vi "CK_CameraParse URL.vi"(10 "Full":bool, 11 "CameraIP":string) -> (0 "cgi string":string, 1 "parameters":T1(array[cluster]), 2 "port":i32, 3 "address":string)   [LabVIEW 2017]
panel:
  # "http://roboRIO-419-FRC.local:5800/?action=stream"
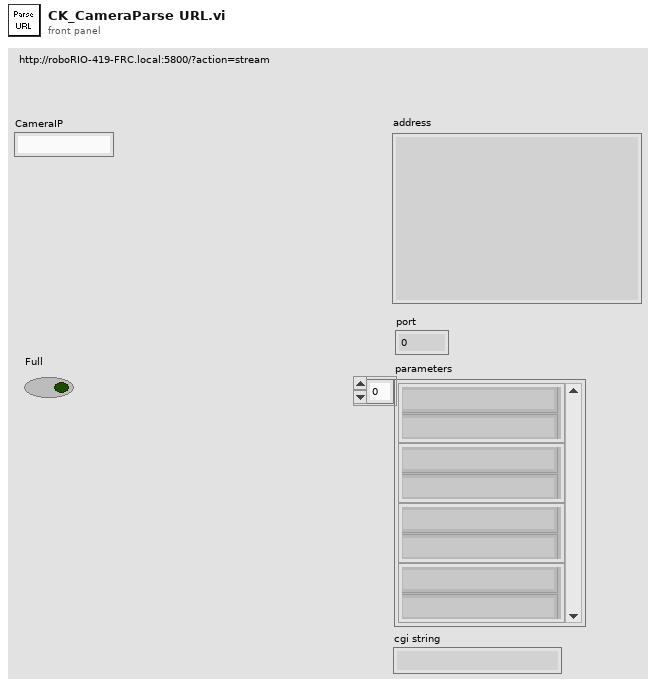
[diagram p1: front panel]
types:
  T1 = cluster{"token string":string, "token string 2":string}[]
  T2 = cluster{"token string":string, "offset past token":i32}
  T3 = cluster{"token string":string, "offset past token":i32}[]
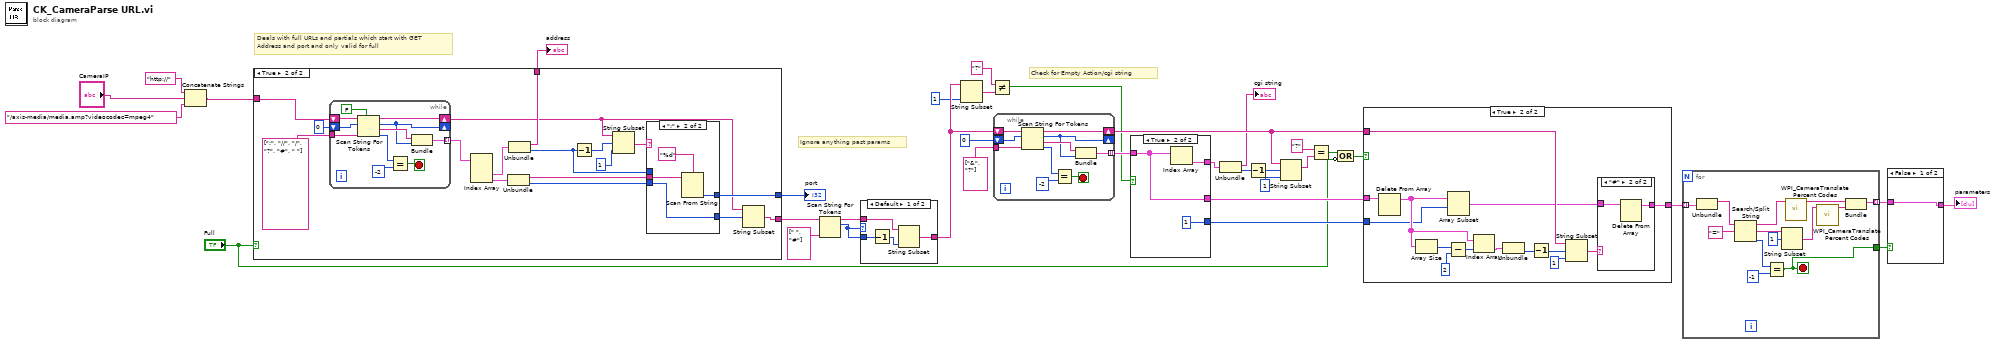
[diagram p0: block diagram]
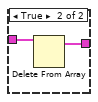
[diagram p4: hidden frame]
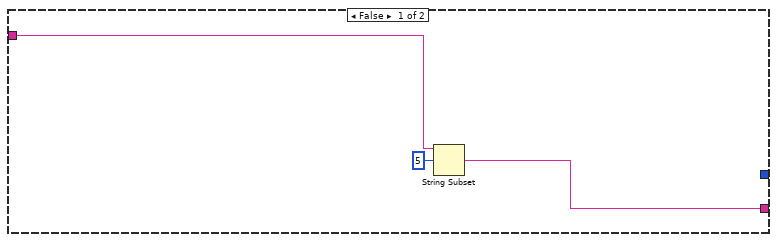
[diagram p5: hidden frame]
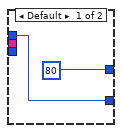
[diagram p6: hidden frame]
diagram:
  # "Check for Empty Action/cgi string"
  # "Ignore anything past params"
  # "Deals with full URLs and partials which start with GET \nAddress and port and only valid for full"
  n1 = Concatenate Strings("http://" ("string"), "CameraIP", "/axis-media/media.amp?videocodec=mpeg4" ("string")) -> (w2:string)
  n2 = case shown="True" "Full" {
    tunnel: [_ w50] -> w35
    tunnel: [_ w49] -> w34
    tunnel: w2 -> [w38 w45]
    tunnel: [w37 w44] -> w16
    frame False {
      n3 = String Subset(string=w38, offset (0)=5) -> (substring=w37:string)  [unwired: 1 in]
    }
    frame True {
      n4 = while {
        tunnel: string[] [":", "//", "/", "?", "#", " "] -> [w72]
        shift-right: [w70] -> w46
        shift-left: w45 -> [w71]
        shift-right: [w63] -> _
        shift-left: 0 ("offset past token") -> [w69]
        tunnel: [w64] -> w53 mode=indexing
        stop <- w67 stop-if-true
        n5 = Scan String For Tokens(5:FALSE ("allow empty tokens? (F)"), 6:w72, 8:w69, 9:w71) -> (0:w65:i32, 1:w66:string, 2:w63:i32, 3:w70:string)  [unwired: 2 in]
        n6 = Equal?(x=w65, y=-2) -> (x = y?=w67:bool)
        n7 = Bundle("token string"=w66, "offset past token"=w63) -> (w64:T2)  [unwired: 1 in]
      }
      n8 = Index Array(array=w53) -> (element #2=w52:T2, element #3=w51:T2)  [unwired: 3 in, 1 out]
      n9 = Unbundle(w51) -> ("token string"=w43:string, "offset past token"=w48:i32)
      n10 = Unbundle(w52) -> ("token string"=w49:string, "offset past token"=w47:i32)
      n11 = Decrement(x=w47) -> (x-1=w41:i32)
      n12 = String Subset(string=w46, offset (0)=w41, length (rest)=1) -> (substring=w40:string)
      n13 = case shown="\":\"" w40 {
        tunnel: w43 -> [_ w61]
        tunnel: [80 w59] -> w50
        tunnel: w48 -> [_ w58]
        tunnel: [w56 w58] -> w39
        tunnel: w47 -> [w56 _]
        frame Default {
        }
        frame ":" {
          n14 = Scan From String(format string="%d", input string=w61) -> (output 1=w59:i32)  [unwired: 3 in, 3 out]
        }
      }
      n15 = String Subset(string=w46, offset (0)=w39) -> (substring=w44:string)  [unwired: 1 in]
    }
  }
  "address" <- w34
  "port" <- w35
  n16 = Scan String For Tokens(6:string[] [" ", "#"], 9:w16) -> (2:w13:i32, 3:w14:string)  [unwired: 4 in, 2 out]
  n17 = case shown="Default" w13 {
    tunnel: w13 -> [w74 _]
    tunnel: [w75 w77] -> w12
    tunnel: w14 -> [w76 w77]
    frame Default {
      n18 = Decrement(x=w74) -> (x-1=w73:i32)
      n19 = String Subset(string=w76, length (rest)=w73) -> (substring=w75:string)  [unwired: 1 in]
    }
    frame -2, -1 {
    }
  }
  n20 = String Subset(string=w12, length (rest)=1 ("length (rest)")) -> (substring=w10:string)  [unwired: 1 in]
  n21 = Not Equal?(x="?" ("format string"), y=w10) -> (x != y?=w7:bool)
  n22 = while {
    tunnel: string[] ["&", "?"] -> [w87]
    shift-right: [w85] -> w27
    shift-left: w12 -> [w86]
    shift-right: [w78] -> _
    shift-left: 0 ("offset past token") -> [w84]
    tunnel: [w79] -> w28 mode=indexing
    stop <- w82 stop-if-true
    n23 = Scan String For Tokens(6:w87, 8:w84, 9:w86) -> (0:w80:i32, 1:w81:string, 2:w78:i32, 3:w85:string)  [unwired: 3 in]
    n24 = Equal?(x=w80, y=-2) -> (x = y?=w82:bool)
    n25 = Bundle("token string"=w81, "offset past token"=w78) -> (w79:T2)  [unwired: 1 in]
  }
  n26 = case shown="True" w7 {
    tunnel: w28 -> [w88 w90]
    tunnel: [_ w91] -> w25
    tunnel: [w88 w90] -> w8
    tunnel: [_ 1] -> w6
    frame False {
    }
    frame True {
      n27 = Index Array(array=w90) -> (element=w91:T2)  [unwired: 1 in]
    }
  }
  n28 = Unbundle(w25) -> ("token string"=→"cgi string":string, "offset past token"=w31:i32)
  n29 = Decrement(x=w31) -> (x-1=w30:i32)
  n30 = String Subset(string=w27, offset (0)=w30, length (rest)=1) -> (substring=w23:string)
  n31 = Equal?(x="?" ("format string"), y=w23) -> (x = y?=w22:bool)
  n32 = Compound Arithmetic op=OR(w22, invert "Full") -> (w21:bool)
  n33 = case shown="True" w21 {
    tunnel: w8 -> [_ w96]
    tunnel: w27 -> [_ w100]
    tunnel: [_ w97] -> w26
    tunnel: w6 -> [_ w92]
    frame False {
    }
    frame True {
      n34 = Delete From Array(array=w96) -> (array with subset deleted=w95:T3)  [unwired: 2 in, 1 out]
      n35 = Array Size(array=w95) -> (size(s)=w94:i32)
      n36 = Array Subset(array=w95, index=w92) -> (w98:T3)  [unwired: 1 in]
      n37 = Subtract(x=w94, y=2) -> (x-y=w105:i32)
      n38 = Index Array(array=w95, index=w105) -> (element=w103:T2)
      n39 = Unbundle(w103) -> ("offset past token"=w104:i32)  [unwired: 1 out]
      n40 = Decrement(x=w104) -> (x-1=w101:i32)
      n41 = String Subset(string=w100, offset (0)=w101, length (rest)=1) -> (substring=w99:string)
      n42 = case shown="\"#\"" w99 {
        tunnel: w98 -> [w106 w108]
        tunnel: [w106 w107] -> w97
        frame "False", Default {
        }
        frame "#" {
          n43 = Delete From Array(array=w108) -> (array with subset deleted=w107:T3)  [unwired: 2 in, 1 out]
        }
      }
    }
  }
  n44 = for {
    tunnel: w26 -> [w121] mode=indexing
    tunnel: [w116] -> w18 mode=indexing
    tunnel: [w113] -> w19
    stop <- w113 stop-if-true
    n45 = Unbundle(w121) -> ("token string"=w117:string)  [unwired: 1 out]
    n46 = Search/Split String(string=w117, search string/char (-)="=" ("format string")) -> (substring before match=w112:string, match + rest of string=w119:string, offset of match=w114:i32)  [unwired: 1 in]
    n47 = Equal?(x=w114, y=-1 ("offset (0)")) -> (x = y?=w113:bool)
    n48 = String Subset(string=w119, offset (0)=1) -> (substring=w109:string)  [unwired: 1 in]
    n49 = call <vilib>:"WPI_CameraTranslate Percent Codes.vi"("String"=w112) -> ("String 2"=w111:string)  [unwired: 10 in]
    n50 = call <vilib>:"WPI_CameraTranslate Percent Codes.vi"("String"=w109) -> ("String 2"=w110:string)  [unwired: 10 in]
    n51 = Bundle("String 2"=w111, "String 2"=w110) -> (w116:cluster{"String 2":string, "String 2":string})  [unwired: 1 in]
  }
  n52 = case shown="False" w19 {
    tunnel: w18 -> [w122 w124]
    tunnel: [w122 w123] -> w17
    frame False {
    }
    frame True {
      n53 = Delete From Array(array=w124) -> (array with subset deleted=w123:cluster{"String 2":string, "String 2":string}[])  [unwired: 2 in, 1 out]
    }
  }
  "parameters" <- w17
